vi "Configure Suspend State.vi"(8 "error in (no error)":errorcluster, 9 "Suspend Impedance (0: Hi-Z)":enum16{"Hi-Z", "Lo-Z"}(ring), 10 "Suspend Voltage (0.0 V)":dbl min=-15.0 max=15.0 step=0.0001 format="%_5g", 11 "VISA resource name":refnum<visa-resource-name>) -> (0 "error out":errorcluster, 3 "VISA resource name out":refnum<visa-resource-name>)   [LabVIEW 2017, in "ADCMT 6240.lvlib"]
doc: "This VI configures the suspend state."
uses:
  ADCMT 6240.lvlib
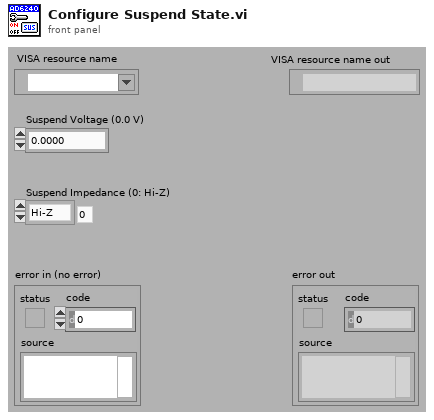
[diagram p1: front panel]
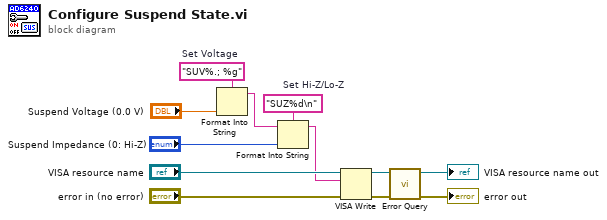
[diagram p0: block diagram]
diagram:
  w3 = "SUZ%d\n"  # Set Hi-Z/Lo-Z
  w9 = "SUV%.; %g"  # Set Voltage
  n1 = Format Into String(format string=w9, "Suspend Voltage (0.0 V)") -> (resulting string=w2:string)  [unwired: 2 in, 1 out]
  n2 = Format Into String(format string=w3, initial string=w2, "Suspend Impedance (0: Hi-Z)") -> (resulting string=w1:string)  [unwired: 1 in, 1 out]
  n3 = VISA Write(VISA resource name="VISA resource name", write buffer=w1, error in (no error)="error in (no error)") -> (VISA resource name out=w8:refnum<visa-resource-name>, error out=w7:errorcluster)  [unwired: 1 out]
  n4 = call "Error Query.vi"("error in (no error)"=w7, "VISA resource name"=w8) -> ("error out"=→"error out":errorcluster, "VISA resource name out"=→"VISA resource name out":refnum<visa-resource-name>)  [unwired: 6 in, 2 out]
